vi "sqlQueryByFigo.vi"(1 "SQL":string, 2 "driver":string="{SQL Server}", 3 "Conditions":string="LuxsharePN='L56SF018-SD-R' AND Eprm_datecode IS NOT NULL", 5 "SheetsName":string="m_HptsVNA_t", 6 "columns":string="*", 7 "DATABASE":string="MESDataCenter", 8 "password":string="querydata", 9 "user id":string="dataquery", 10 "Server":string="DG-MESDB.luxshare.com.cn", 11 "Timeout":i32=30) -> (0 "查询数据":string[][](array[string]), 4 "query status":bool)   [LabVIEW 2011]
panel:
  out "SQL语句":string
  out "数据库连接字符串":string
  out "GetString":string
  in  "ADODB._Recordset":refnum<k7>
  in  "ADODB._Connection":refnum<k7>
  # "输入"
  # "输出"
  # "driver={SQL Server};Server=DG-MESDB.luxshare.com.cn;user id=dataquery;password=querydata;DATABASE=MESDataCenter"
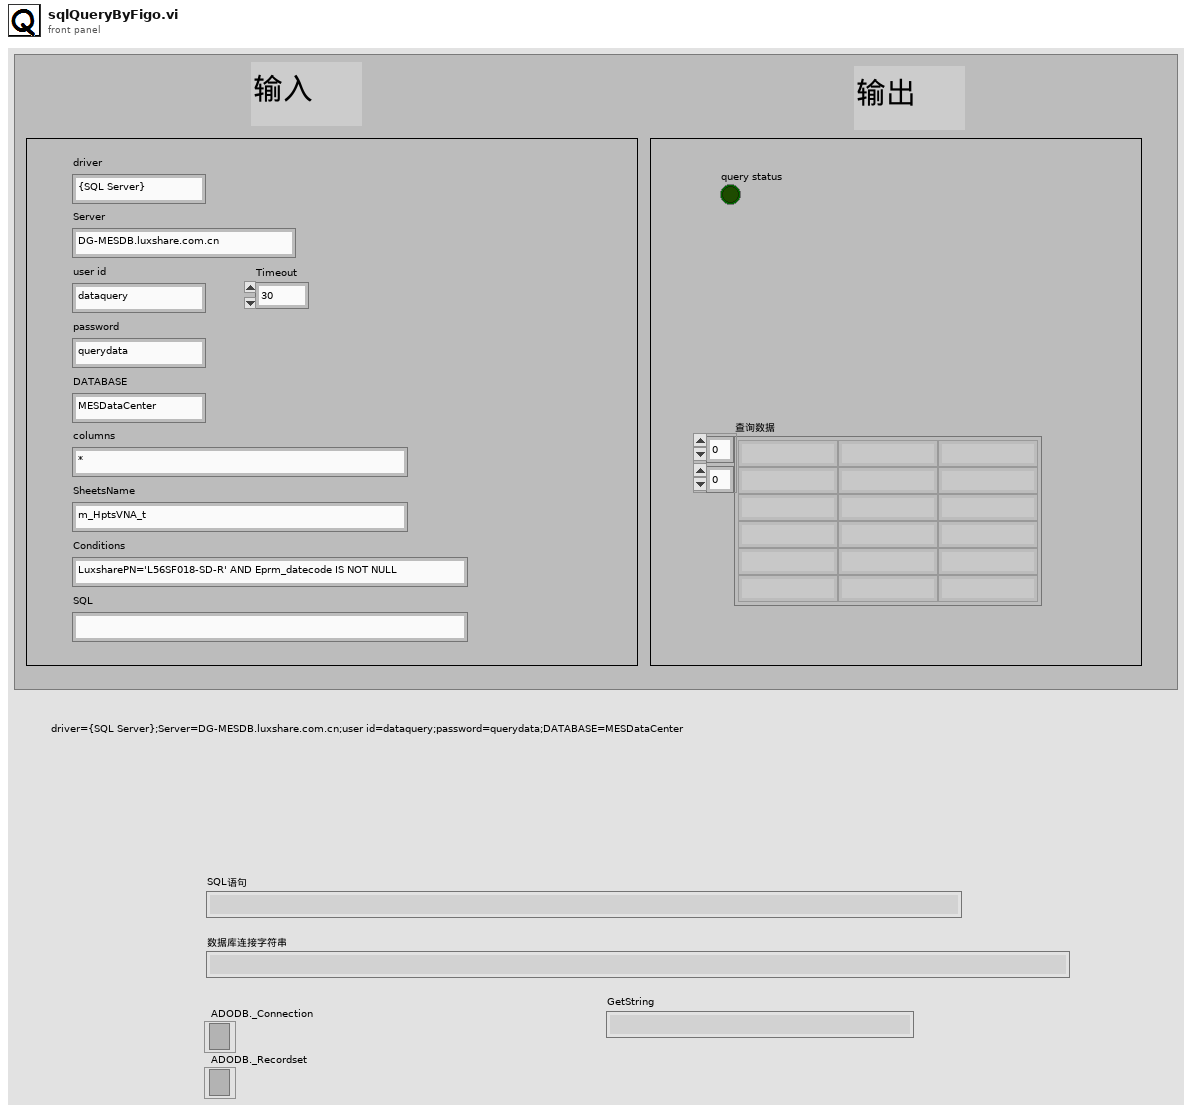
[diagram p1: front panel]
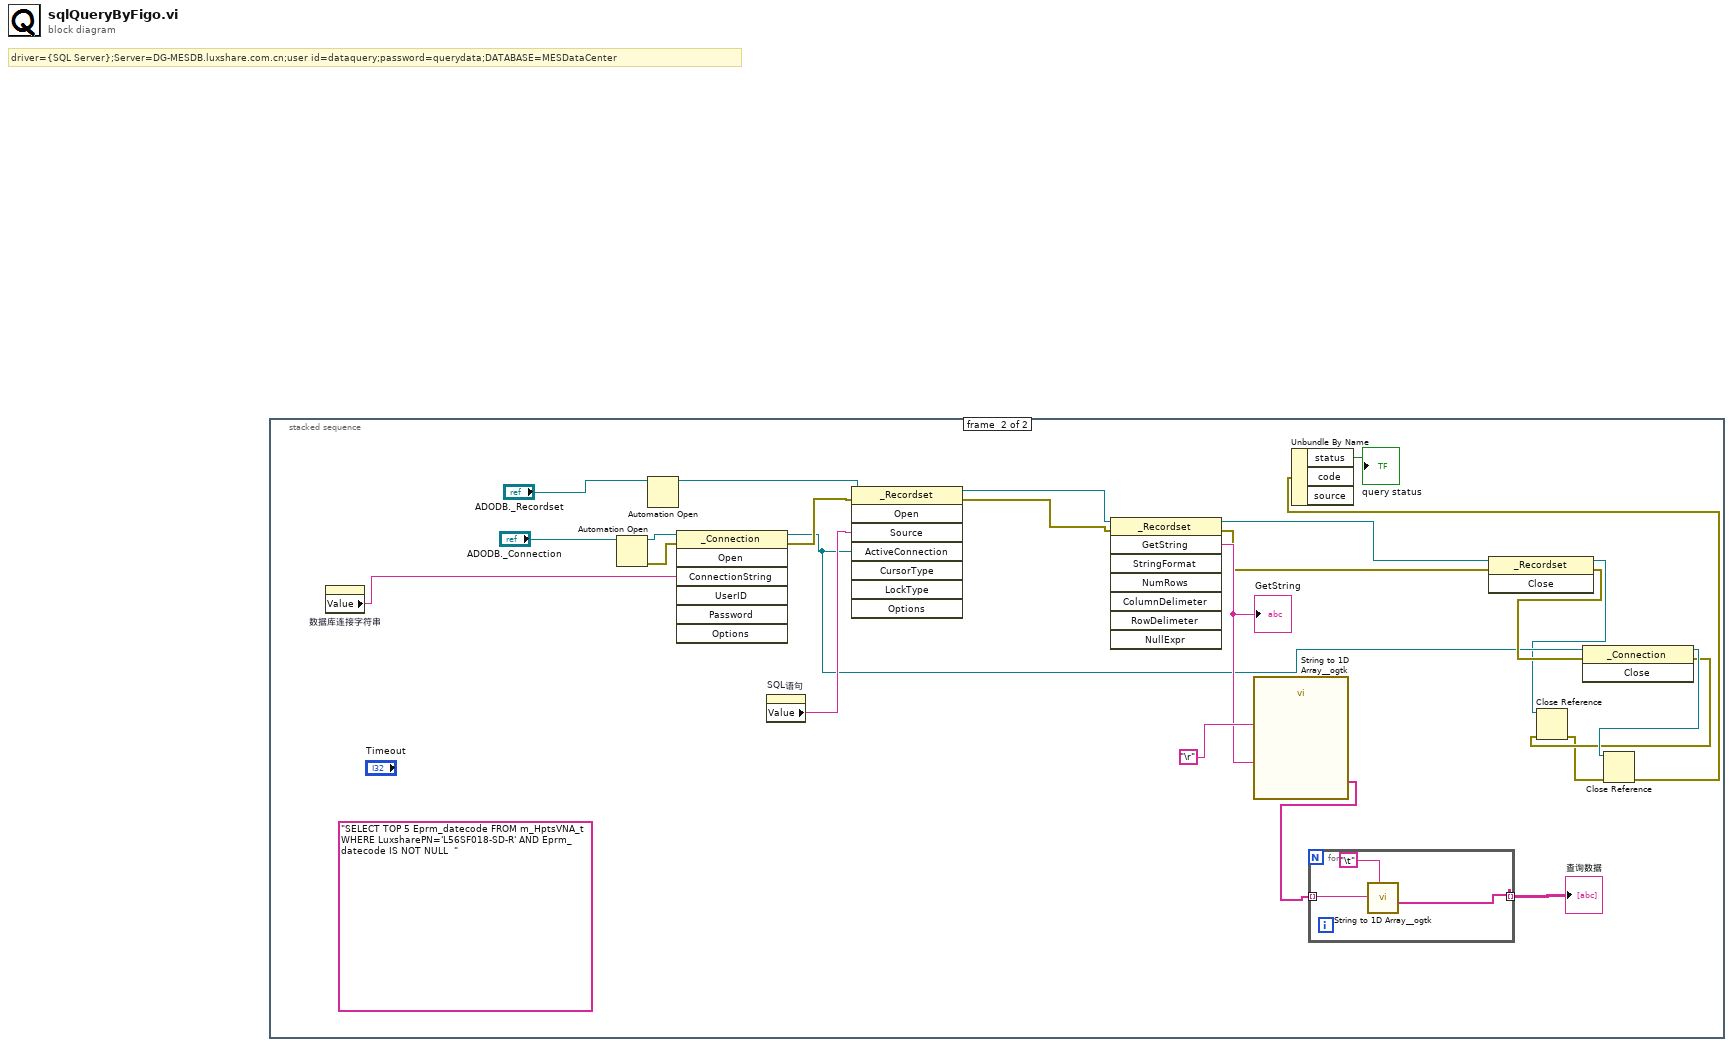
[diagram p0: block diagram]
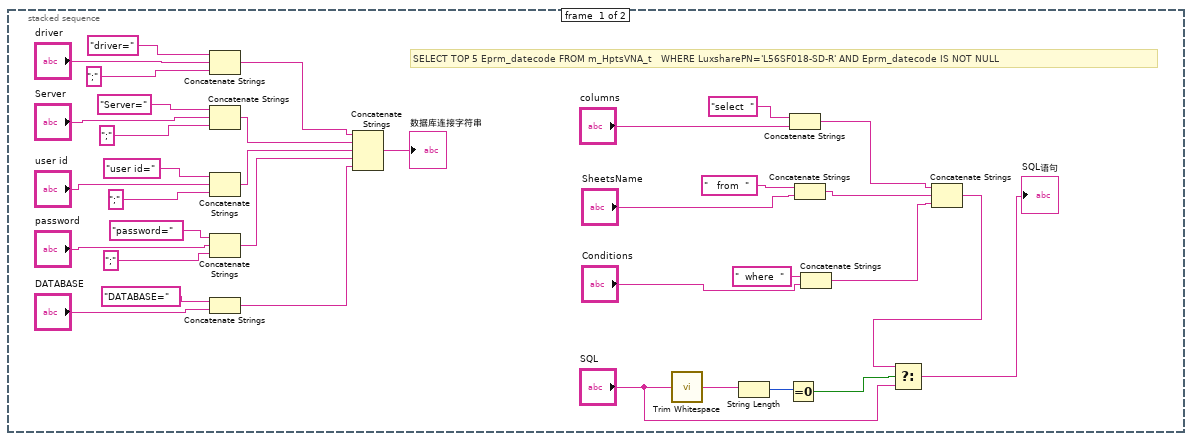
[diagram p2: hidden frame]
diagram:
  # "driver={SQL Server};Server=DG-MESDB.luxshare.com.cn;user id=dataquery;password=querydata;DATABASE=MESDataCenter"
  n1 = stacked-sequence {
    frame #0 {
      # "SELECT TOP 5 Eprm_datecode FROM m_HptsVNA_t   WHERE LuxsharePN='L56SF018-SD-R' AND Eprm_datecode IS NOT NULL"
      n2 = Concatenate Strings("driver=" ("字符串"), "driver", ";" ("字符串")) -> (w21:string)
      n3 = Concatenate Strings("Server=" ("字符串"), "Server", ";" ("字符串")) -> (w20:string)
      n4 = Concatenate Strings("user id=" ("字符串"), "user id", ";" ("字符串")) -> (w19:string)
      n5 = Concatenate Strings("password=" ("字符串"), "password", ";" ("字符串")) -> (w18:string)
      n6 = Concatenate Strings("DATABASE=" ("字符串"), "DATABASE") -> (w17:string)
      n7 = Concatenate Strings(w21, w20, w19, w18, w17) -> (→"数据库连接字符串":string)
      n8 = call <vilib>:"Trim Whitespace.vi"("string"="SQL") -> ("trimmed string"=w6:string)  [unwired: 1 in]
      n9 = String Length(string=w6) -> (length=w5:i32)
      n10 = Equal To 0?(x=w5) -> (x = 0?=w4:bool)
      n11 = Concatenate Strings("select  " ("字符串"), "columns") -> (w9:string)
      n12 = Concatenate Strings("   from  " ("字符串"), "SheetsName") -> (w8:string)
      n13 = Concatenate Strings("  where  " ("字符串"), "Conditions") -> (w7:string)
      n14 = Concatenate Strings(w9, w8, w7) -> (w3:string)
      n15 = Select(t=w3, s=w4, f="SQL") -> (s? t:f=→"SQL语句":string)
    }
    frame #1 {
      (unwired) "SELECT TOP 5 Eprm_datecode FROM m_HptsVNA_t   WHERE LuxsharePN='L56SF018-SD-R' AND Eprm_datecode IS NOT NULL  "
      n16 = property on="数据库连接字符串" class="Str"() -> ("Value"=w41:string)  [unwired: 2 in, 2 out]
      n17 = Automation Open(Automation Refnum="ADODB._Connection") -> (Automation Refnum=w43:refnum<k7>, error out=w42:errorcluster)  [unwired: 3 in]
      n18 = Automation Open(Automation Refnum="ADODB._Recordset") -> (Automation Refnum=w50:refnum<k7>)  [unwired: 3 in, 1 out]
      n19 = invoke class="_Connection" method="Open"(reference=w43, error in=w42, "ConnectionString"=w41) -> (reference out=w44:refnum<k7>, error out=w51:errorcluster)  [unwired: 4 in, 5 out]
      n20 = property on="SQL语句" class="Str"() -> ("Value"=w46:string)  [unwired: 2 in, 2 out]
      n21 = invoke class="_Recordset" method="Open"(reference=w50, error in=w51, "Source"=w46, "ActiveConnection"=w44) -> (reference out=w45:refnum<k7>, error out=w59:errorcluster)  [unwired: 4 in, 6 out]
      n22 = invoke class="_Recordset" method="GetString"(reference=w45, error in=w59) -> (reference out=w53:refnum<k7>, error out=w54:errorcluster, "GetString"=w55:string)  [unwired: 6 in, 5 out]
      "GetString" <- w55
      n23 = call <userlib>:"String to 1D Array__ogtk.vi"("delimiter (Tab)"="\r", "string"=w55) -> ("Array of Strings"=w58:string[])  [unwired: 9 in]
      n24 = for {
        tunnel: [w62] -> w57 mode=indexing
        tunnel: w58 -> [w60] mode=indexing
        n25 = call <userlib>:"String to 1D Array__ogtk.vi"("delimiter (Tab)"="\t", "string"=w60) -> ("Array of Strings"=w62:string[])  [unwired: 9 in]
      }
      "查询数据" <- w57
      n26 = invoke class="_Recordset" method="Close"(reference=w53, error in=w54) -> (reference out=w40:refnum<k7>, error out=w47:errorcluster)  [unwired: 1 in, 1 out]
      n27 = invoke class="_Connection" method="Close"(reference=w44, error in=w47) -> (reference out=w39:refnum<k7>, error out=w38:errorcluster)  [unwired: 1 in, 1 out]
      n28 = Close Reference(reference=w40, error in (no error)=w38) -> (error out=w37:errorcluster)
      n29 = Close Reference(reference=w39, error in (no error)=w37) -> (error out=w36:errorcluster)
      n30 = Unbundle By Name(w36) -> ("status"=→"query status":bool)  [unwired: 2 out]
    }
  }
